vi "Test Process Returns Error When Requesting Top Level Context.vi"(8 "error in (no error)":errorcluster, 11 "Process Test In":refnum<class "Process Test.lvclass">) -> (0 "error out":errorcluster, 3 "Process Test Out":refnum<class "Process Test.lvclass">)   [LabVIEW 2020, in "Process Test.lvclass"]
uses:
  Process Test.lvclass
  C:/Program Files (x86)/National Instruments/LabVIEW 2020/vi.lib/Asteme/LUnit/Test Case.lvclass
  Framework/Process/Process.lvclass/Process.ctl
  <vilib>/Asteme/LUnit/Test Case.lvclass/Test Case.ctl
  <vilib>/Asteme/LUnit/LUnit Assertion Result.lvclass/LUnit Assertion Result.ctl
  Framework/Process/Public/Get Lifecycle State.vi
  <vilib>/Asteme/LUnit/Palette/Fail.vi
  <vilib>/Asteme/LUnit/Palette/Pass.vi
  <vilib>/Asteme/LUnit/Set Assertion Type.vi
  <vilib>/Asteme/LUnit/Variant to string.vi
  Framework/Process/Private/SubVIs/Wait for finish.vi
  Framework/Process/Protected/Messaging/Enqueue Message.vi
  Framework/Process/Private/SubVIs/Set Lifecycle State.vi
  <vilib>/Utility/error.llb/Clear Errors.vi
  <vilib>/Asteme/LUnit/Add test result.vi
  <vilib>/Asteme/LUnit/LUnit Write Passed.vi
  <vilib>/Asteme/LUnit/LUnit Get Test Case.vi
  <vilib>/Asteme/LUnit/LUnit Write Message.vi
  <vilib>/Asteme/LUnit/LUnit Write Description.vi
  <vilib>/Asteme/LUnit/LUnit Write Assertion Type.vi
  <vilib>/AdvancedString/1D String Array to Delimited String.vi
  <vilib>/Asteme/LUnit/Read Test Case Name.vi
  <vilib>/Utility/error.llb/Error Cluster From Error Code.vi
  <vilib>/Asteme/LUnit/Assertion Result/LUnit Get Test Name.vi
  <vilib>/Utility/Data Type/Get Type Information.vi
  <vilib>/Utility/LVClass/Get LV Class Name.vi
  Framework/Application/Application.lvclass
  <vilib>/Asteme/LUnit/LUnit Assertion Result.lvclass
  Framework/Process/Process.lvclass
  <vilib>/Asteme/LUnit/Test Case.lvclass
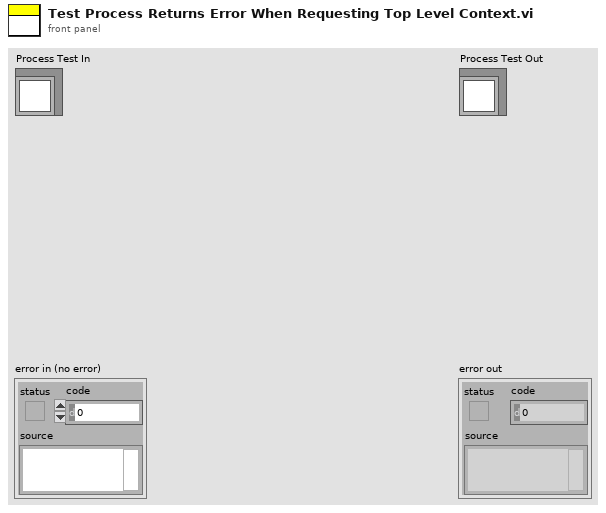
[diagram p1: front panel]
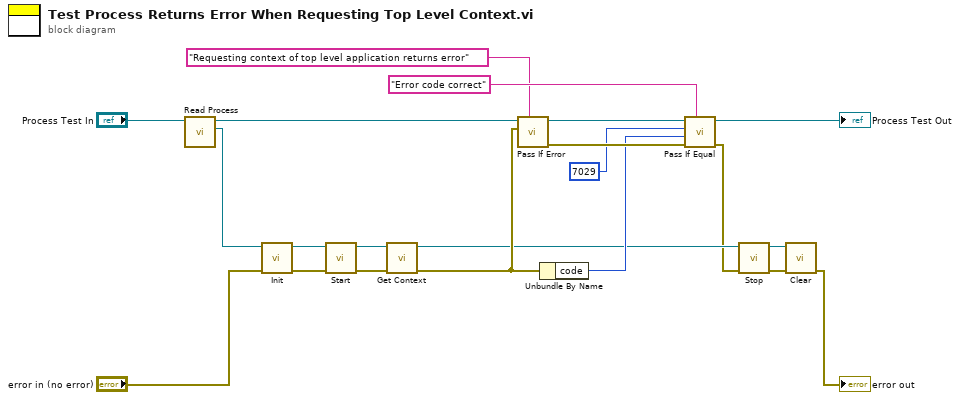
[diagram p0: block diagram]
diagram:
  n1 = call "Read Process.vi"("Process Test in"="Process Test In") -> ("Process.lvclass"=w11:refnum<class "Process.lvclass">, "Process Test out"=w20:refnum<class "Process Test.lvclass">)  [unwired: 8 in, 1 out]
  n2 = call-dynamic "Init.vi"("error in (no error)"="error in (no error)", "Process In"=w11) -> ("error out"=w7:errorcluster, "Process Out"=w9:refnum<class "Process.lvclass">)  [unwired: 8 in]
  n3 = call "Start.vi"("error in (no error)"=w7, "Process In"=w9) -> ("error out"=w6:errorcluster, "Process Out"=w8:refnum<class "Process.lvclass">)  [unwired: 8 in]
  n4 = call "Get Context.vi"("error in (no error)"=w6, "Process In"=w8) -> ("error out"=w16:errorcluster, "Process Out"=w5:refnum<class "Process.lvclass">)  [unwired: 7 in, 1 out]
  n5 = call <vilib>:"Pass If Error.vi"("Description"="Requesting context of top level application returns error", "Assert error"=w16, "Test Case In"=w20) -> ("error out"=w17:errorcluster, "Test Case Out"=w19:refnum<class "Process Test.lvclass">)  [unwired: 7 in]
  n6 = Unbundle By Name(w16) -> ("code"=w14:i32)
  n7 = call <vilib>:"Pass If Equal.vi"("Description"="Error code correct", "error in (no error)"=w17, "Actual"=w14, "Expected"=7029 ("code"), "Test Case In"=w19) -> ("error out"=w2:errorcluster, "Test Case Out"=→"Process Test Out":refnum<class "Process Test.lvclass">)  [unwired: 5 in]
  n8 = call "Stop.vi"("error in (no error)"=w2, "Process In"=w5) -> ("error out"=w3:errorcluster, "Process Out"=w4:refnum<class "Process.lvclass">)  [unwired: 7 in, 1 out]
  n9 = call-dynamic "Clear.vi"("error in (no error)"=w3, "Process In"=w4) -> ("error out"=→"error out":errorcluster)  [unwired: 8 in, 1 out]
